vi "Display Balance Status.vi"(8 "error in (no error)":errorcluster, 10 "Max Exceeded? In":bool, 11 "New Balance":dbl) -> (0 "error out":errorcluster, 2 "Max Exceeded? Out":bool, 3 "Messages":T1)   [LabVIEW 2026]
uses:
  controls/Data.ctl
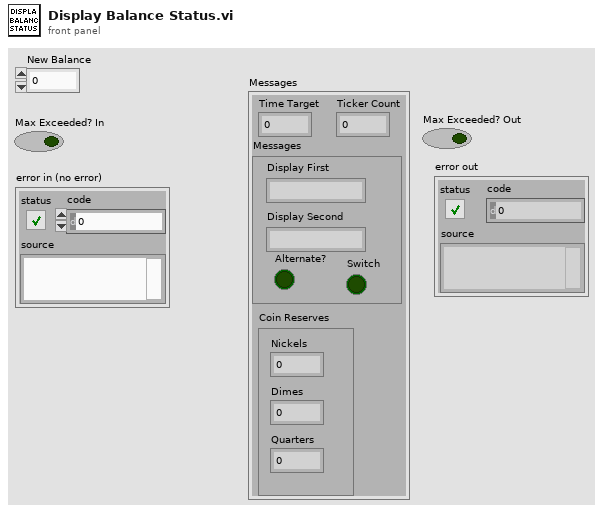
[diagram p1: front panel]
types:
  T1 = typedef "Data.ctl" = cluster{"Time Target":dbl, "Messages":cluster{"Display First":string, "Display Second":string, "Alternate?":bool, "Switch":bool}, "Ticker Count":dbl, "Coin Reserves":cluster{"Nickels":dbl, "Dimes":dbl, "Quarters":dbl}}
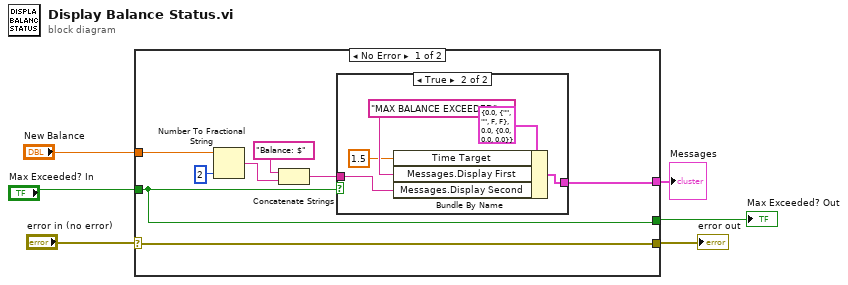
[diagram p0: block diagram]
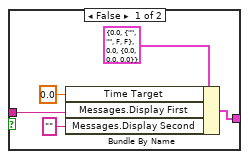
[diagram p2: hidden frame]
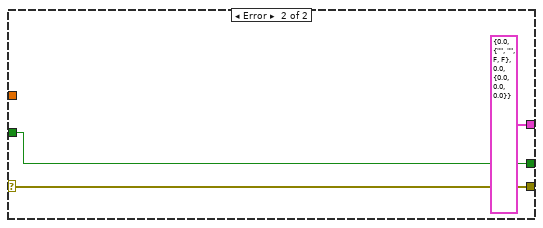
[diagram p3: hidden frame]
diagram:
  n1 = case shown="No Error" "error in (no error)" {
    selector: "error in (no error)" -> [w14 w27]
    tunnel: "Max Exceeded? In" -> [w13 w26]
    tunnel: [w7 T1 {"Time Target"=0.0, "Messages"={"Display First"="", "Display Second"="", "Alternate?"=FALSE, "Switch"=FALSE}, "Ticker Count"=0.0, "Coin Reserves"={"Nickels"=0.0, "Dimes"=0.0, "Quarters"=0.0}} ("Data")] -> w1
    tunnel: "New Balance" -> [w9 _]
    tunnel: [w14 w27] -> w3
    tunnel: [w13 w26] -> w2
    frame No Error {
      n2 = Number To Fractional String(number=w9, precision (6)=i16 2) -> (F-format string=w11:string)  [unwired: 2 in]
      n3 = Concatenate Strings("Balance: $" ("Message"), w11) -> (w8:string)
      n4 = case shown="True" w13 {
        tunnel: [w17 w23] -> w7
        tunnel: w8 -> [w16 w21]
        frame False {
          n5 = Bundle By Name(cluster=T1 {"Time Target"=0.0, "Messages"={"Display First"="", "Display Second"="", "Alternate?"=FALSE, "Switch"=FALSE}, "Ticker Count"=0.0, "Coin Reserves"={"Nickels"=0.0, "Dimes"=0.0, "Quarters"=0.0}} ("Data"), "Time Target"=0.0, "Messages.Display First"=w16, "Messages.Display Second"="") -> (w17:T1)
        }
        frame True {
          n6 = Bundle By Name(cluster=T1 {"Time Target"=0.0, "Messages"={"Display First"="", "Display Second"="", "Alternate?"=FALSE, "Switch"=FALSE}, "Ticker Count"=0.0, "Coin Reserves"={"Nickels"=0.0, "Dimes"=0.0, "Quarters"=0.0}} ("Data"), "Time Target"=1.5, "Messages.Display First"="MAX BALANCE EXCEEDED", "Messages.Display Second"=w21) -> (w23:T1)
        }
      }
    }
    frame Error {
    }
  }
  "error out" <- w3
  "Max Exceeded? Out" <- w2
  "Messages" <- w1
